vi "Update Thrust Dots.vi"(11 "Ship in":refnum<class "Ship.lvclass">) -> (3 "Ship out":refnum<class "Ship.lvclass">)   [LabVIEW 2021, in "Ship.lvclass"]
uses:
  Ship.lvclass
  Ship.lvclass/Ship.ctl
  Element/Element.lvclass
  Motion/Motion.lvclass
  Thrust Dot/Thrust Dot.lvclass
  Control State/Control State.lvclass
  Re-use Libraries/Vector 2D/Vector 2D.lvclass
  Math/Vec2.ctl
  Math/Math.lvlib
panel:
  in  "Point":T1={"x"=50.0, "y"=50.0}
  in  "y":dbl=0.25 format="%#_13g"
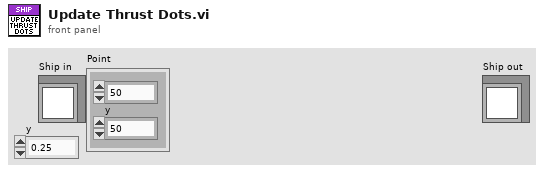
[diagram p1: front panel]
types:
  T1 = typedef "Math.lvlib/Vec2.ctl" = cluster{"x":sgl, "y":sgl}
  T2 = typedef "Control State.lvclass/Button State.ctl" = enum16{"Undefined", "Pressed", "Released", "Held", "Not Held"}
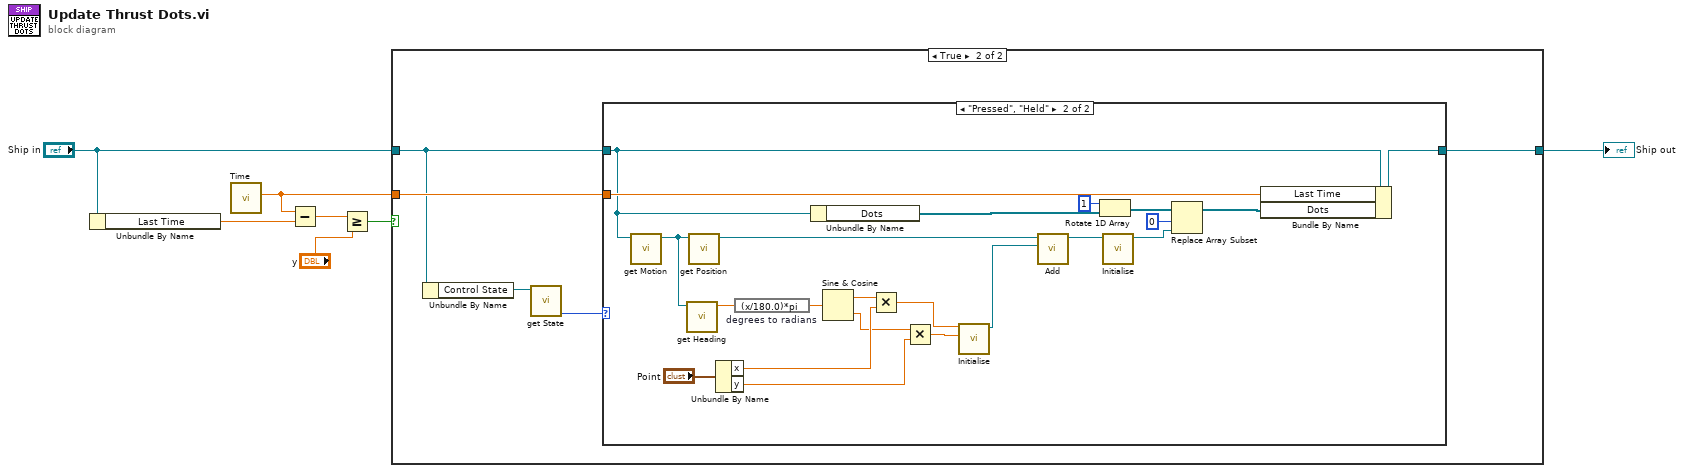
[diagram p0: block diagram]
diagram:
  n1 = Unbundle By Name("Ship in") -> ("Last Time"=w7:sgl)
  n2 = call "Time.vi"() -> ("Time [s]"=w1:sgl)  [unwired: 10 in, 1 out]
  n3 = Subtract(x=w1, y=w7) -> (x-y=w6:sgl)
  n4 = Greater Or Equal?(x=w6, y="y") -> (x >= y?=w4:bool)
  n5 = case shown="True" w4 {
    tunnel: "Ship in" -> [w8 w11]
    tunnel: w1 -> [_ w13]
    tunnel: [w8 w12] -> w2
    frame False {
    }
    frame True {
      n6 = Unbundle By Name(w11) -> ("Control State"=w10:refnum<class "Control State.lvclass">)
      n7 = call "get State.vi"("Control State in"=w10) -> ("Thrust"=w9:T2)  [unwired: 6 in, 4 out]
      n8 = case shown="\"Pressed\", \"Held\"" w9 {
        tunnel: w13 -> [_ w36]
        tunnel: [w14 w35] -> w12
        tunnel: w11 -> [w14 w28]
        frame Default {
        }
        frame "Pressed", "Held" {
          n9 = call "get Motion.vi"("Element in"=w28) -> ("Motion"=w27:refnum<class "Motion.lvclass">)  [unwired: 10 in]
          n10 = call "get Heading.vi"("Motion in"=w27) -> ("Heading [deg]"=w26:sgl)  [unwired: 10 in]
          n11 = call "get Position.vi"("Motion in"=w27) -> ("Displacement"=w16:refnum<class "Vector 2D.lvclass">)  [unwired: 10 in]
          n12 = Unbundle By Name("Point") -> ("x"=w22:sgl, "y"=w20:sgl)
          n13 = expression code="(x/180.0)*pi" "degrees to radians"(w26) -> (w24:sgl)
          n14 = Unbundle By Name(w28) -> ("Dots"=w34:refnum<class "Thrust Dot.lvclass">[])
          n15 = Sine & Cosine(0:w24) -> (1:w23:sgl, 2:w21:sgl)
          n16 = Multiply(x=w23, y=w22) -> (x*y=w19:sgl)
          n17 = Multiply(x=w21, y=w20) -> (x*y=w18:sgl)
          n18 = call "Initialise.vi"("y"=w18, "x"=w19) -> ("Vector 2D out"=w17:refnum<class "Vector 2D.lvclass">)  [unwired: 9 in]
          n19 = call "Add.vi"("B"=w17, "A"=w16) -> ("A+B"=w15:refnum<class "Vector 2D.lvclass">)  [unwired: 9 in]
          n20 = Rotate 1D Array(1:w34, 2:1 ("n")) -> (0:w32:refnum<class "Thrust Dot.lvclass">[])
          n21 = call "Initialise.vi"("Position"=w15) -> ("Thrust Dot out"=w29:refnum<class "Thrust Dot.lvclass">)  [unwired: 10 in]
          n22 = Replace Array Subset(array=w32, new element=w29, index=0) -> (w31:refnum<class "Thrust Dot.lvclass">[])
          n23 = Bundle By Name(cluster=w28, "Last Time"=w36, "Dots"=w31) -> (w35:refnum<class "Ship.lvclass">)
        }
      }
    }
  }
  "Ship out" <- w2
